vi "integal_pickup_sequence .vi"(0 "store_pos":u8, 1 "pick_pos":u8=45, 2 "target_ir_l":dbl, 3 "target_ir_r":dbl, 4 "precision":dbl) -> ()   [LabVIEW 2017]
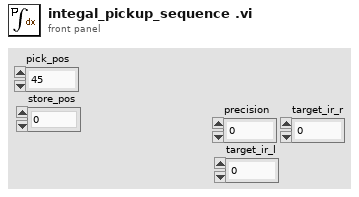
[diagram p1: front panel]
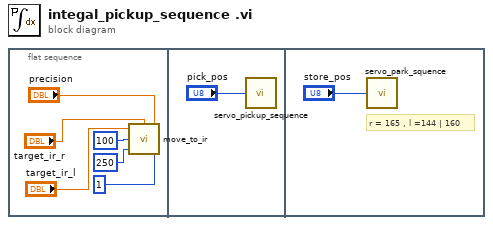
[diagram p0: block diagram]
diagram:
  n1 = flat-sequence {
    frame #0 {
      n2 = call "move_to_ir.vi"("step"=1, "precision"="precision", "target_ir_r"="target_ir_r", "samples"=250, "delay_after"=u32 100, "target_ir_l"="target_ir_l") -> ()
    }
    frame #1 {
      n3 = call "servo_pickup_sequence.vi"("servo 3"="pick_pos") -> ()
    }
    frame #2 {
      # "r = 165 , l =144 | 160"
      n4 = call "servo_park_squence.vi"("servo 3"="store_pos") -> ()
    }
  }
